vi "configure piezo and pockelscontrol for galvo.vi"() -> (0 "error out":errorcluster, 3 "task out":refnum<k21>)   [LabVIEW 2012]
uses:
  <vilib>/DAQmx/write.llb/DAQmx Write (Analog 2D DBL NChan NSamp).vi
  GFG/GFGstringGet.vi
  GFG/GFGfpRefGet.vi
  GFG/GFGnumericGet.vi
  GFG/GFGbooleanGet.vi
  <vilib>/DAQmx/create/channels.llb/DAQmx Create Channel (AO-Voltage-Basic).vi
  <vilib>/DAQmx/miscellaneous.llb/DAQmx Fill In Error Info.vi
  GFG/GFG library.lvlib
  <resource>/objmgr/daqmx.rc
panel:
  out "pockels cell control":dbl[](graph)
  out "piezo control":dbl[](graph)
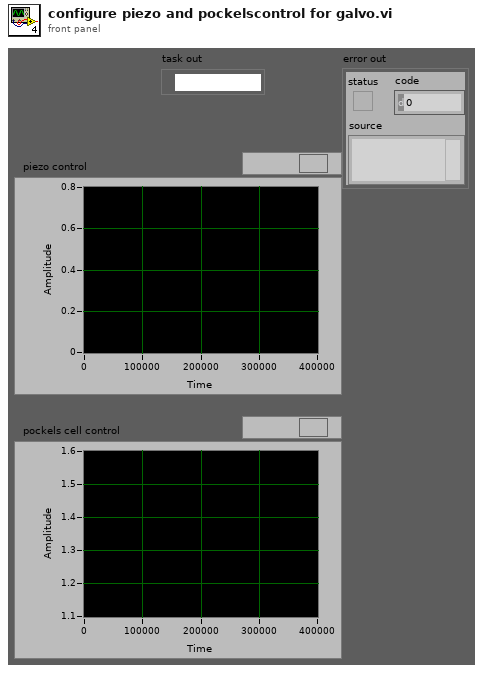
[diagram p1: front panel]
types:
  T1 = enum8{"Enabled", "Disabled", "Disabled and Grayed Out"}
  T2 = cluster{"WaveformChartRef":refnum<vi>, "DigitalRef":refnum<vi>, "ArrayRef":refnum<vi>, "TabControlRef":refnum<vi>, "EnumRef":refnum<vi>, "RingRef":refnum<vi>, "BooleanRef":refnum<vi>, "KnobRef":refnum<vi>, "SlideRef":refnum<vi>, "PathRef":refnum<vi>, "StringRef":refnum<vi>, "ComboBox":refnum<vi>, "WaveformGraphRef":refnum<vi>}
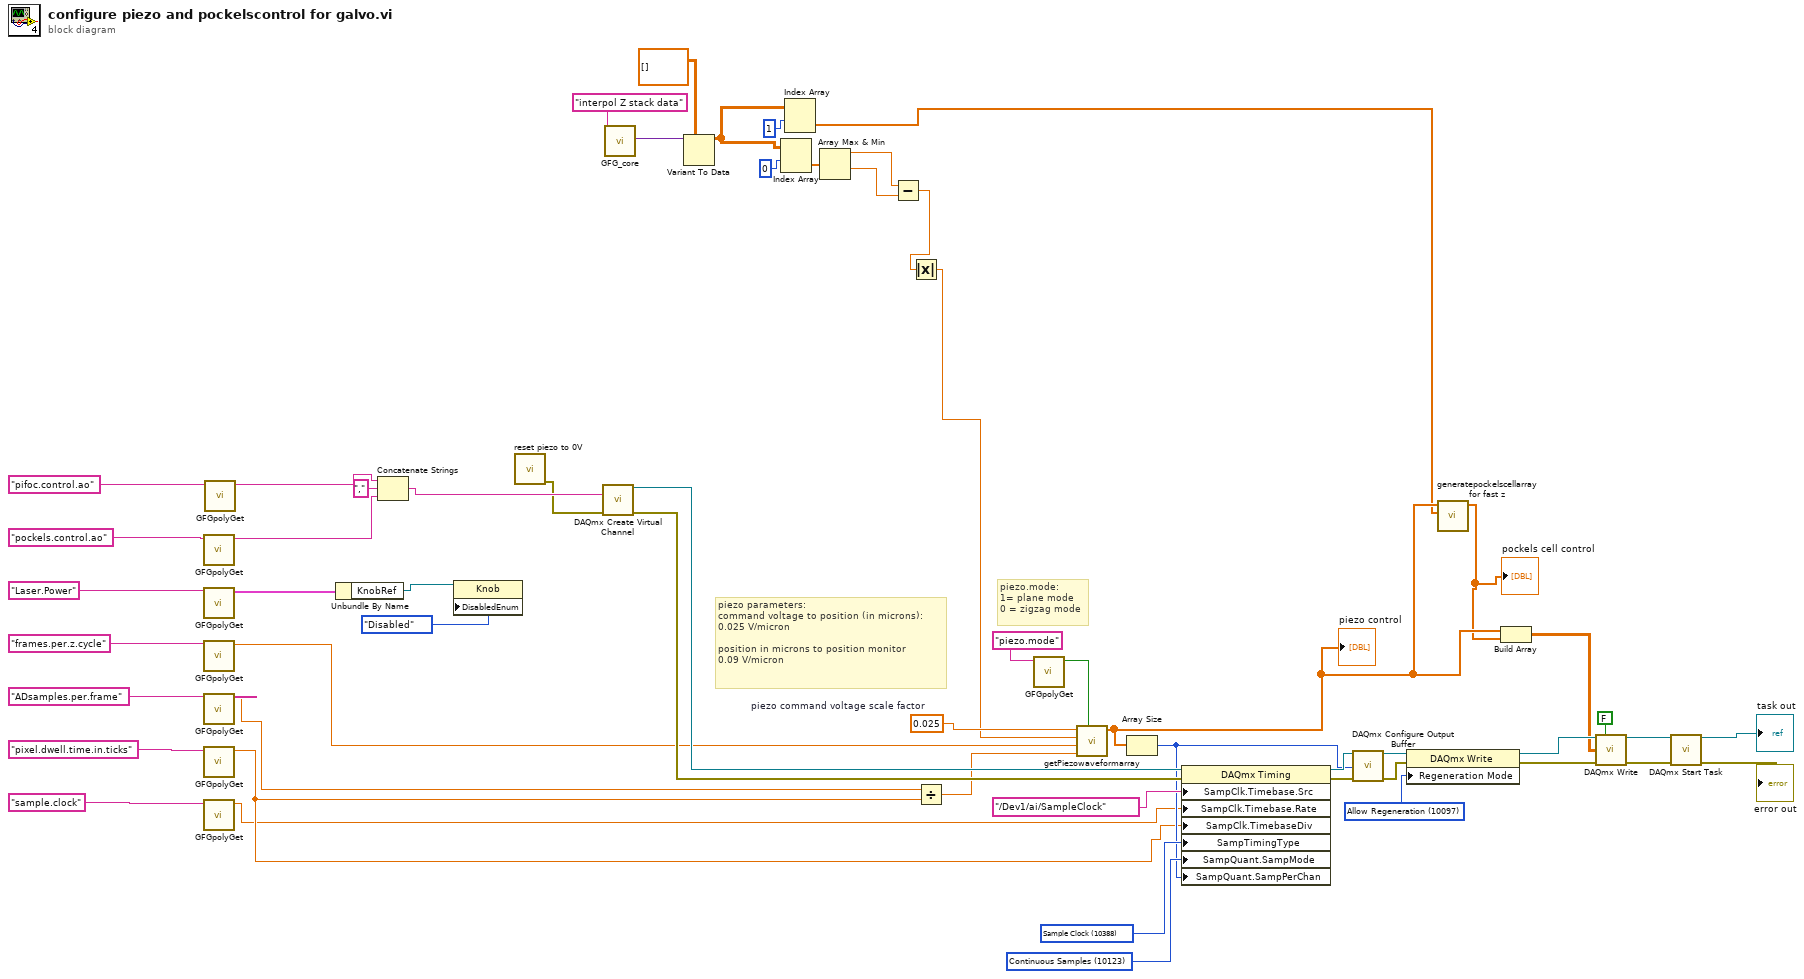
[diagram p0: block diagram]
diagram:
  w32 = 0.025  # piezo command voltage scale factor
  w38 = 10388 items=["Sample Clock"=10388, "Burst Handshake"=12548, "Handshake"=10389, "Implicit"=10451, "On Demand"=10390, "Change Detection"=12504, "Pipelined Sample Clock"=14668] ("SampTimingType")
  w46 = 10097 items=["Allow Regeneration"=10097, "Do Not Allow Regeneration"=10158] ("RegenMode")
  w37 = 10123 items=["Finite Samples"=10178, "Continuous Samples"=10123] ("sample mode")
  # "piezo.mode: \n1= plane mode\n0 = zigzag mode"
  # "piezo parameters:\ncommand voltage to position (in microns):\n0.025 V/micron\n\nposition in microns to position monitor\n0.09 V/micron"
  n1 = call-poly "GFGpolyGet.vi"("Variable Name in"="pockels.control.ao" ("Tag in")) -> ("String"=w52:string)  [unwired: 10 in]
  n2 = call-poly "GFGpolyGet.vi"("Variable Name in"="Laser.Power") -> ("output cluster"=w50:T2)  [unwired: 9 in, 1 out]
  n3 = call-poly "GFGpolyGet.vi"("Variable Name in"="frames.per.z.cycle" ("Tag in")) -> ("Numeric"=w22:dbl)  [unwired: 9 in, 1 out]
  n4 = call-poly "GFGpolyGet.vi"("Variable Name in"="ADsamples.per.frame" ("Tag in")) -> ("Numeric"=w24:dbl)  [unwired: 9 in, 1 out]
  n5 = call-poly "GFGpolyGet.vi"("Variable Name in"="pixel.dwell.time.in.ticks" ("Tag in")) -> ("Numeric"=w26:dbl)  [unwired: 9 in, 1 out]
  n6 = call-poly "GFGpolyGet.vi"("Variable Name in"="sample.clock" ("Tag in")) -> ("Numeric"=w4:dbl)  [unwired: 9 in, 1 out]
  n7 = call-poly "GFGpolyGet.vi"("Variable Name in"="pifoc.control.ao") -> ("String"=w53:string)  [unwired: 10 in]
  n8 = Unbundle By Name(w50) -> ("KnobRef"=w49:refnum<vi>)
  n9 = Concatenate Strings(w53, "," ("string"), w52) -> (w28:string)
  n10 = property class="Knob"(reference=w49, "DisabledEnum"=T1."Disabled" ("Disabled")) -> ()  [unwired: 1 in, 2 out]
  n11 = call "reset piezo to 0V.vi"() -> ("error out"=w3:errorcluster)  [unwired: 11 in]
  n12 = call-poly <vilib>:"DAQmx Create Virtual Channel.vi"("physical channels"=w28, "error in"=w3) -> ("task out"=w39:refnum<k21>, "error out"=w41:errorcluster)  [unwired: 12 in]
  n13 = call "GFG_core.vi"("Variable Name in"="interpol Z stack data") -> ("Variant Out"=w20:variant)  [unwired: 12 in, 6 out]
  n14 = Variant To Data(type=dbl[][] [] ("Interpolated Data"), Variant=w20) -> (data=w18:dbl[][])  [unwired: 1 in, 1 out]
  n15 = Index Array(array=w18, index (row)=0 ("disabled index (col)")) -> (element=w17:dbl[])  [unwired: 1 in]
  n16 = Index Array(array=w18, index (row)=1 ("disabled index (col)")) -> (element=w7:dbl[])  [unwired: 1 in]
  n17 = Array Max & Min(array=w17) -> (max value=w16:dbl, min value=w15:dbl)  [unwired: 2 out]
  n18 = Subtract(x=w16, y=w15) -> (x-y=w14:dbl)
  n19 = Absolute Value(x=w14) -> (abs(x)=w9:dbl)
  n20 = Divide(x=w24, y=w26) -> (x/y=w31:dbl)
  n21 = call-poly "GFGpolyGet.vi"("Variable Name in"="piezo.mode" ("Tag in")) -> ("Boolean"=w10:bool)  [unwired: 10 in]
  n22 = call "getPiezowaveformarray.vi"("planes or zigzag"=w10, "pixel.num"=w31, "frames.per.z.cycle"=w22, "total.z.distance"=w9, "piezo scale factor"=w32) -> ("Array"=w8:dbl[])  [unwired: 6 in]
  "piezo control" <- w8
  n23 = Array Size(array=w8) -> (size(s)=w30:i32)
  n24 = property class="DAQmx Timing"(reference=w39, error in=w41, "SampClk.Timebase.Src"=tag "/Dev1/ai/SampleClock" ("Clock Source"), "SampClk.Timebase.Rate"=w4, "SampClk.TimebaseDiv"=w26, "SampTimingType"=w38, "SampQuant.SampMode"=w37, "SampQuant.SampPerChan"=w30) -> (reference out=w35:refnum<k21>, error out=w42:errorcluster)
  n25 = call <vilib>:"DAQmx Configure Output Buffer.vi"("task/channels in"=w35, "buffer size (in samples per channel)"=w30, "error in"=w42) -> ("task out"=w47:refnum<k21>, "error out"=w45:errorcluster)  [unwired: 11 in]
  n26 = property class="DAQmx Write"(reference=w47, error in=w45, "Regeneration Mode"=w46) -> (reference out=w43:refnum<k21>, error out=w44:errorcluster)
  n27 = call "generatepockelscellarray for fast z.vi"("interpolated pockels cell data"=w7, "piezo control"=w8) -> ("pockelscellarray"=w6:dbl[])  [unwired: 9 in]
  "pockels cell control" <- w6
  n28 = Build Array(w8, w6) -> (w29:dbl[][])
  n29 = call-poly <vilib>:"DAQmx Write.vi"("task/channels in"=w43, "auto start"=FALSE, "data"=w29, "error in"=w44) -> ("task out"=w34:refnum<k21>, "error out"=w36:errorcluster)  [unwired: 9 in, 1 out]
  n30 = call <vilib>:"DAQmx Start Task.vi"("task/channels in"=w34, "error in"=w36) -> ("task out"=→"task out":refnum<k21>, "error out"=→"error out":errorcluster)  [unwired: 12 in]
